vi "FG MC VISA Resource.vi"(2 "FG Action (Read)":T1, 3 "MC VISA resource in":refnum<visa-resource-name>="ASRL1::INSTR") -> (1 "MC VISA resource out":refnum<visa-resource-name>="ASRL1::INSTR")   [LabVIEW 2009]
uses:
  Actions for FG's.ctl
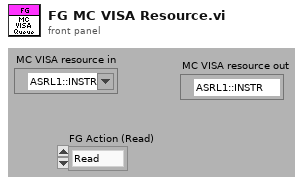
[diagram p1: front panel]
types:
  T1 = typedef "Actions for FG's.ctl" = enum16{"Read", "Write"}
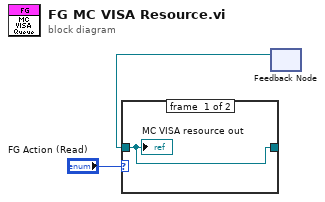
[diagram p0: block diagram]
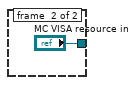
[diagram p2: hidden frame]
diagram:
  n1 = feedback #1() -> (w1:refnum<visa-resource-name>)  [unwired: 1 in]
  n2 = case shown="\"Read\", Default" "FG Action (Read)" {
    tunnel: [w4 "MC VISA resource in"] -> w2
    tunnel: w1 -> [w4 _]
    frame #0 {
      "MC VISA resource out" <- w4
    }
    frame #1 {
    }
  }
